vi "RF-BME280-Logger.vi"() -> ()   [LabVIEW 2018]
uses:
  Program Files (x86)/National Instruments/LabVIEW 2018/examples/Instrument IO/Serial/support/Serial - XON-XOFF Characters.ctl
  Program Files (x86)/National Instruments/LabVIEW 2018/examples/Instrument IO/Serial/support/Serial - ASCII Characters.ctl
  Program Files (x86)/National Instruments/LabVIEW 2018/examples/Instrument IO/Serial/support/Serial - Settings.ctl
  <vilib>/Instr/_visa.llb/VISA Configure Serial Port (Instr).vi
panel:
  out "log path":path
  out "error out":errorcluster
  in  "VISA resource name":refnum<visa-resource-name>="COM1"
  out "Response":string
  in  "Stop":bool
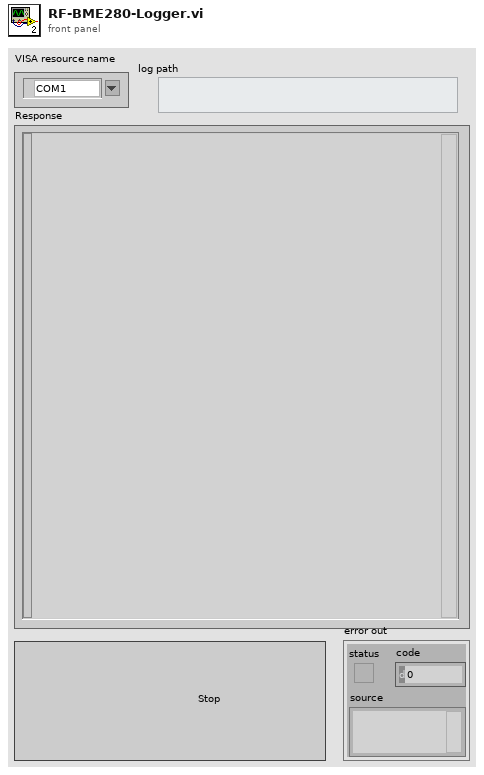
[diagram p1: front panel]
types:
  T1 = typedef "Serial - Settings.ctl" = cluster{"baud rate":u32, "data bits":u16, "parity":enum16{"None", "Odd", "Even", "Mark", "Space"}, "stop bits":u16, "flow control":u16}
  T2 = typedef "Serial - XON-XOFF Characters.ctl" = cluster{"XON":T3, "XOFF":T3}
  T3 = typedef "Serial - ASCII Characters.ctl" = enum16{"NUL", "SOH", "STX", "ETX", "EOT", "ENQ", "ACK", "BEL", "BS", "HT", "LF", "VT", "FF", "CR", "SO", "SI", "DLE", "DC1", "DC2", "DC3", "DC4", "NAK", "SYN", "ETB", "CAN", "EM", "SUB", "ESC", "FS", "GS", "RS", "US", "SP", "!", "\"", "#", "$", "%", "&", "'", "(", ")", "*", "+", ",", "- (-)", ".", "/", "0", "1", "2", "3", "4", "5", "6", "7", "8", "9", ":", ";", "<", "=", ">", "?", "@", "A", "B", "C", "D", "E", "F", "G", "H", "I", "J", "K", "L", "M", "N", "O", "P", "Q", "R", "S", "T", "U", "V", "W", "X", "Y", "Z", "[", "\\", "]", "^", "_", "`", "a", "b", "c", "d", "e", "f", "g", "h", "i", "j", "k", "l", "m", "n", "o", "p", "q", "r", "s", "t", "u", "v", "w", "x", "y", "z", "{", "|", "}", "~"}
  T4 = enum16{"open", "replace", "create", "open or create", "replace or create", "replace or create with confirmation"}
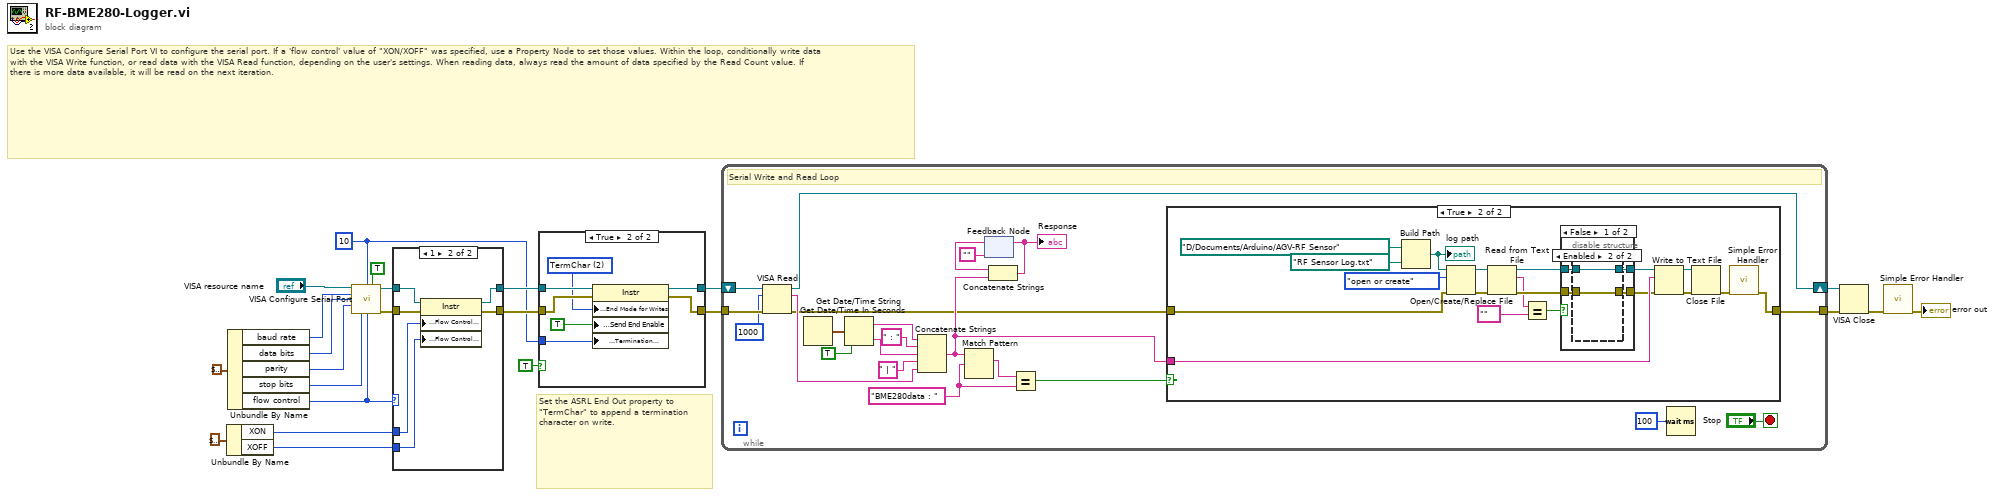
[diagram p0: block diagram]
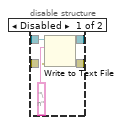
[diagram p5: hidden frame]
diagram:
  w2 = u8 10 ("Termination Character")
  # "Set the ASRL End Out property to \"TermChar\" to append a termination character on write."
  # "Use the VISA Configure Serial Port VI to configure the serial port. If a 'flow control' value of \"XON/XOFF\" was specified, use a Property Node to set those values. Within the loop, conditionally write data with the VISA Write function, or read data with the VISA Read function, depending on the user's settings. When reading data, always read the amount of data specified by the Read Count value. If there is more data available, it will be read on the next iteration."
  n1 = Unbundle By Name(T2 {"XON"=enum."DC1", "XOFF"=enum."DC3"} ("XON/XOFF Characters")) -> ("XON"=w9:T3, "XOFF"=w8:T3)
  n2 = Unbundle By Name(T1 {"baud rate"=115200, "data bits"=8, "parity"=enum."None", "stop bits"=10, "flow control"=0} ("Serial Settings")) -> ("baud rate"=w16:u32, "data bits"=w17:u16, "parity"=w18:enum16{"None", "Odd", "Even", "Mark", "Space"}, "stop bits"=w19:u16, "flow control"=w10:u16)
  n3 = call-poly "VISA Configure Serial Port"("VISA resource name"="VISA resource name", "termination char\n(0xA = '\\n' = LF)"=w2, "Enable Termination\nChar (T)"=TRUE ("End Read on Termination Character?"), "baud rate (9600)"=w16, "data bits (8)"=w17, "parity (0:none)"=w18, "stop bits (10: 1 bit)"=w19, "flow control (0:none)"=w10) -> ("VISA resource name out"=w20:refnum<visa-resource-name>, "error out"=w21:errorcluster)  [unwired: 2 in, 4 out]
  n4 = case shown="1" w10 {
    tunnel: [w24 w31] -> w7
    tunnel: [w25 w30] -> w5
    tunnel: w21 -> [w24 w29]
    tunnel: w20 -> [w25 w28]
    tunnel: w9 -> [_ w27]
    tunnel: w8 -> [_ w26]
    frame Default {
    }
    frame 1 {
      n5 = property class="Instr"(reference=w28, error in=w29, "Serial Settings:Flow Control XON Character"=w27, "Serial Settings:Flow Control XOFF Character"=w26) -> (reference out=w30:refnum<visa-resource-name>, error out=w31:errorcluster)
    }
  }
  n6 = case shown="True" TRUE ("End Write on Termination Character?") {
    tunnel: w5 -> [w32 w40]
    tunnel: w7 -> [w33 w39]
    tunnel: [w32 w38] -> w4
    tunnel: [w33 w37] -> w6
    tunnel: w2 -> [_ w35]
    frame False {
    }
    frame True {
      w36 = u16 2 items=["None", "LastBit", "TermChar", "Break"] ("Serial Settings:Serial End Mode for Writes")
      n7 = property class="Instr"(reference=w40, error in=w39, "Serial Settings:End Mode for Writes"=w36, "Message Based Settings:Send End Enable"=TRUE, "Message Based Settings:Termination Character"=w35) -> (reference out=w38:refnum<visa-resource-name>, error out=w37:errorcluster)
    }
  }
  n8 = while {
    shift-right: [w42] -> w11
    shift-left: w4 -> [w62]
    tunnel: w6 -> [w61]
    tunnel: [w41] -> w12
    stop <- "Stop" stop-if-true
    w46 = "BME280data : "
    # "Serial Write and Read Loop"
    n9 = VISA Read(VISA resource name=w62, byte count=u32 1000 ("Read Count"), error in (no error)=w61) -> (VISA resource name out=w42:refnum<visa-resource-name>, read buffer=w48:string, error out=w43:errorcluster)  [unwired: 1 out]
    n10 = Get Date/Time In Seconds() -> (seconds since 1Jan1904=w54:timestamp)
    n11 = Get Date/Time String(seconds (now)=w54, want seconds? (F)=TRUE) -> (date string=w52:string, time string=w50:string)  [unwired: 1 in]
    n12 = Concatenate Strings(w52, " : " ("string"), w50, " | " ("string"), w48) -> (w45:string)
    n13 = Match Pattern(string=w45, regular expression=w46) -> (match substring=w47:string)  [unwired: 1 in, 3 out]
    n14 = feedback #1("") -> (w57:string)
    n15 = Concatenate Strings(w57, w45) -> (w55:string)
    "Response" <- w55
    n16 = feedback-in #1(w55) -> ()
    n17 = Equal?(x=w47, y=w46) -> (x = y?=w44:bool)
    n18 = case shown="True" w44 {
      tunnel: w45 -> [_ w82]
      tunnel: w43 -> [w63 w65]
      tunnel: [w63 w64] -> w41
      frame False {
      }
      frame True {
        n19 = Build Path(base path=path "D:/Documents/Arduino/AGV-RF Sensor", name or relative path=path "RF Sensor Log.txt" ("default name")) -> (appended path=w78:path)
        "log path" <- w78
        n20 = Open/Create/Replace File(file path (use dialog)=w78, error in=w65, operation (0:open)=T4."open or create") -> (refnum out=w74:refnum<file>, error out=w73:errorcluster)  [unwired: 3 in, 1 out]
        n21 = Read from Text File(file (use dialog)=w74, error in=w73) -> (refnum out=w72:refnum<file>, text=w68:string, error out=w70:errorcluster)  [unwired: 2 in, 1 out]
        n22 = Equal?(x=w68, y="" ("string")) -> (x = y?=w66:bool)
        n23 = case shown="False" w66 {
          tunnel: w72 -> [w86 w95]
          tunnel: [w85 w95] -> w71
          tunnel: w70 -> [w84 w94]
          tunnel: [w83 w94] -> w69
          frame False {
            n24 = disable-structure shown="Enabled" {
              disable-tunnel: w86 -> [w90 w93]
              disable-tunnel: [w89 w93] -> w85
              disable-tunnel: w84 -> [w88 w92]
              disable-tunnel: [w87 w92] -> w83
              frame Disabled {
                n25 = Write to Text File(file (use dialog)=w90, text="\n", error in=w88) -> (refnum out=w89:refnum<file>, error out=w87:errorcluster)  [unwired: 1 in, 1 out]
              }
              frame Enabled {
              }
            }
          }
          frame True {
          }
        }
        n26 = Write to Text File(file (use dialog)=w71, text=w82, error in=w69) -> (refnum out=w76:refnum<file>, error out=w75:errorcluster)  [unwired: 1 in, 1 out]
        n27 = Close File(refnum=w76, error in=w75) -> (error out=w80:errorcluster)  [unwired: 1 out]
        n28 = call <vilib>:"Simple Error Handler.vi"("error in (no error)"=w80) -> ("error out"=w64:errorcluster)  [unwired: 4 in, 4 out]
      }
    }
    n29 = Wait (ms)(milliseconds to wait=u32 100) -> ()  [unwired: 1 out]
  }
  n30 = VISA Close(VISA resource name=w11, error in (no error)=w12) -> (error out=w13:errorcluster)
  n31 = call <vilib>:"Simple Error Handler.vi"("error in (no error)"=w13) -> ("error out"=→"error out":errorcluster)  [unwired: 1 in, 7 out]
